vi "Vision.vi"() -> ()   [LabVIEW 2021]
doc: "Main VI for the vision algorithm. Shows camera footage and extracts ball and plate position, that are then written on the myRIO microcontroller to be used by other programs. Refresh rate of coordinates is 17ms"
uses:
  <vilib>/Platform/TimedLoop/XDataNode/timing_clust.ctl
  <vilib>/Platform/TimedLoop/XDataNode/nitl_modes.ctl
  <vilib>/Platform/TimedLoop/XDataNode/wakeup.ctl
  <vilib>/Platform/TimedLoop/XDataNode/XDataNode.xnode
  <vilib>/Platform/TimedLoop/XDataNode/XDNodeRunTimeDep.lvlib
panel:
  in  "Exposure::Value":dbl=1.0 min=0.0625 max=32.0
  in  "Exposure::Mode":u32(ring)=2 items=["Auto"=1, "Manual"=2]
  in  "error in":errorcluster
  out "Ball Coordinates":sgl[](array[numeric])
  out "Plate coordinates":sgl[](array[numeric])
  out "error out":errorcluster
  out "Frame Rate":dbl
  in  "Stop (F)":bool
  out "Image Out":T1(plugin-control)
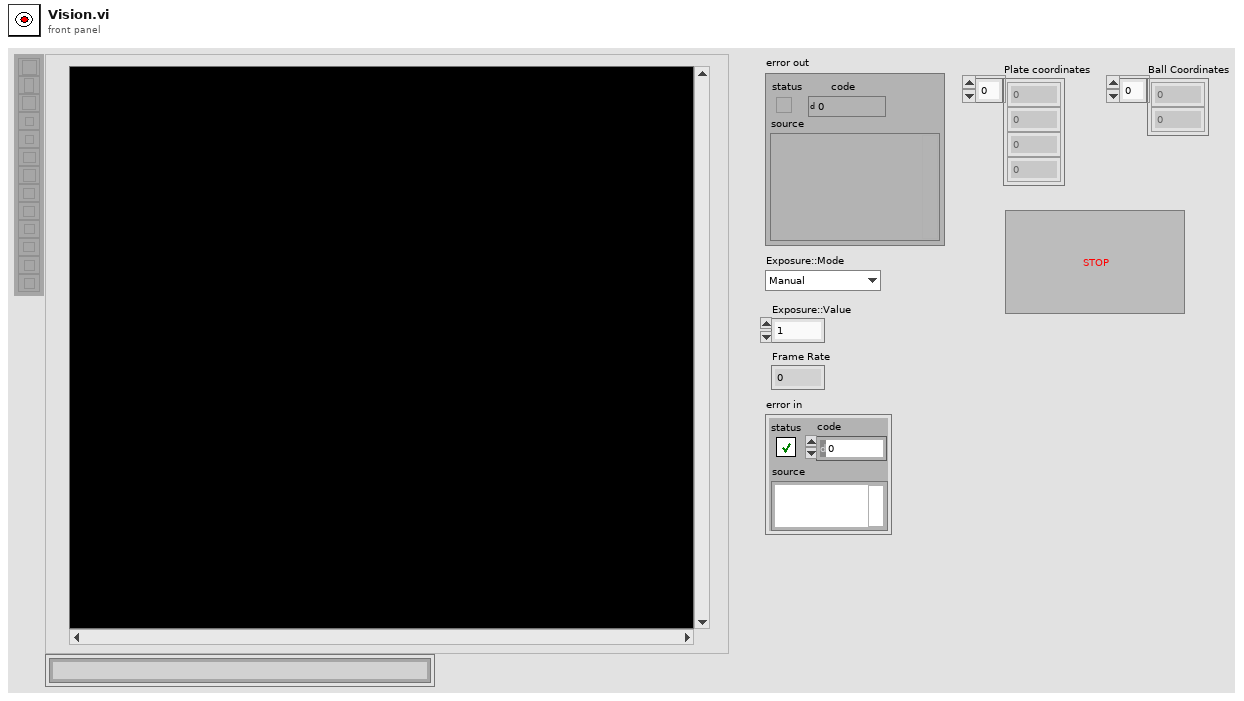
[diagram p1: front panel]
types:
  T1 = typedef "IMAQ Image.ctl" = refnum<image>
  T2 = typedef "XDNodeRunTimeDep.lvlib/timing_clust.ctl" = cluster{"Expected End [f-1]":u64, "Actual End [f-1]":u64, "Finished Late? [f-1]":bool, "Expected End [i-1]":u64, "Actual End [i-1]":u64, "Finished Late? [i-1]":bool, "Expected Start [i]":u64, "Actual Start [i]":u64, "Expected Start [f]":u64, "Actual Start [f]":u64, "Source Name":string, "Structure Name":string, "Period":i64, "Deadline":i64, "Offset":i64, "Start":i64, "Priority":i32, "Timeout":i32, "Mode":T3, "Wakeup Reason":T4, "Error":errorcluster, "Source Type":string, "Secondary Source Type":string, "Global End Time":u64, "Global Start Time":u64, "Frame Duration":u64, "Iteration Duration":u64, "Assigned CPU":i32, "I/O Scan Engine Mode":u32}
  T3 = typedef "XDNodeRunTimeDep.lvlib/nitl_modes.ctl" = enum32{"No Change", "Process missed periods, maintain original phase", "Discard missed periods, maintain original phase", "Process missed periods, ignore original phase", "Discard missed periods, ignore original phase"}
  T4 = typedef "XDNodeRunTimeDep.lvlib/wakeup.ctl" = enum32{"Normal", "Aborted", "Asynchronous wakeup", "Timing source error", "Timed loop error", "Timeout"}
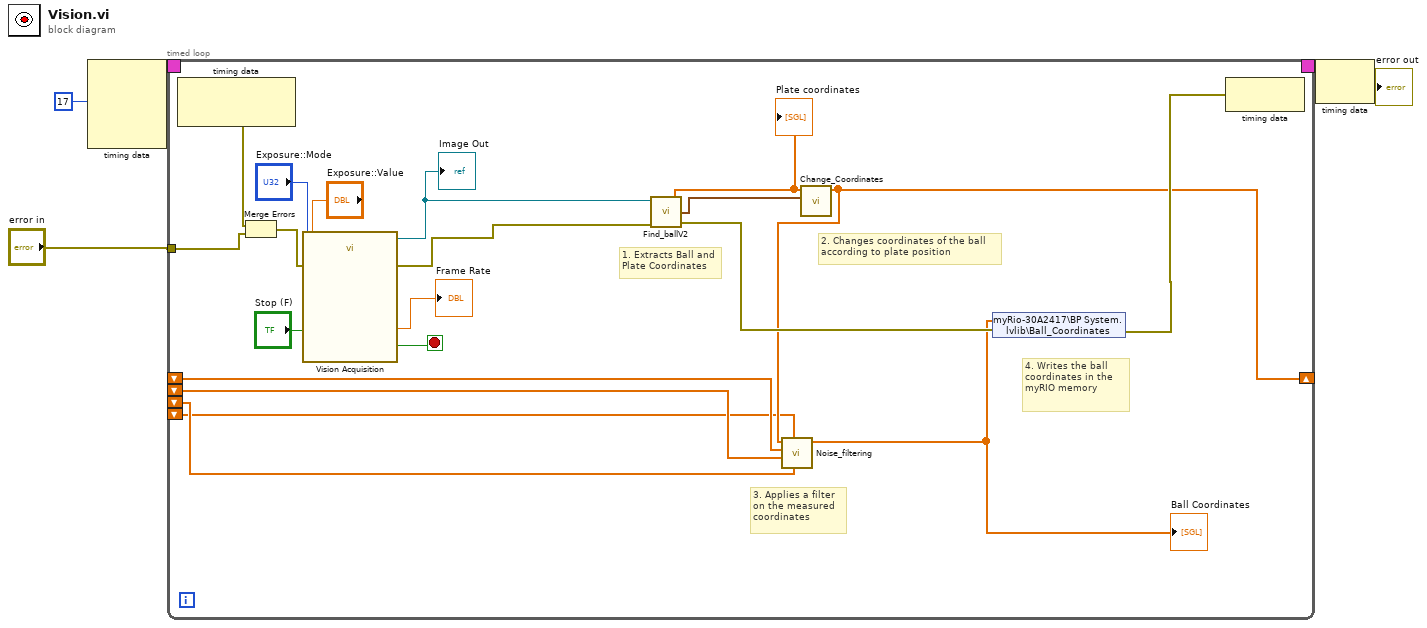
[diagram p0: block diagram]
diagram:
  n1 = node-c288(i64 17 ("Period")) -> (w5:T2)  [unwired: 3 in]
  n2 = timed-loop {
    timing: w5 -> [_]
    timing-out: [_] -> w4
    tunnel: "error in" -> [w15]
    shift-right: [w11] -> _
    shift-left: _ -> [w10]
    shift-left: _ -> [w9]
    shift-left: _ -> [w8]
    shift-left: _ -> [w7]
    stop <- w24 stop-if-true
    # "4. Writes the ball coordinates in the myRIO memory"
    # "2. Changes coordinates of the ball\naccording to plate position"
    # "1. Extracts Ball and\nPlate Coordinates"
    # "3. Applies a filter\non the measured \ncoordinates"
    n3 = node-c288() -> (w16:errorcluster)  [unwired: 1 in, 1 out]
    n4 = Merge Errors(w16, w15) -> (w14:errorcluster)
    n5 = call "Vision Acquisition"("Exposure::Mode"="Exposure::Mode", "Exposure::Value"="Exposure::Value", "Stop (F)"="Stop (F)", "error in"=w14) -> ("Image Out"=w22:T1, "Frame Rate"=→"Frame Rate":dbl, "Stopped"=w24:bool, "error out"=w18:errorcluster)  [unwired: 20 in]
    "Image Out" <- w22
    n6 = call "Find_ballV2.vi"("Image In"=w22, "error in"=w18) -> ("Plate coordinates"=w20:sgl[], "Ball Coordinates"=w21:cluster{"x":sgl, "y":sgl}, "error out"=w19:errorcluster)  [unwired: 2 in, 1 out]
    "Plate coordinates" <- w20
    n7 = call "Change_Coordinates.vi"("Ball Coordinates"=w21, "Plate coordinates"=w20) -> ("Array"=w11:sgl[])  [unwired: 9 in]
    n8 = call "Noise_filtering.vi"("Array 3"=w8, "Array in"=w7, "Array 4"=w9, "Array 5"=w10, "Array 6"=w11) -> ("Array out"=w6:dbl[])  [unwired: 6 in]
    "Ball Coordinates" <- w6
    n9 = shared-variable "myRio-30A2417\\BP System.lvlib\\Ball_Coordinates"(w6, error in=w19) -> (error out=w17:errorcluster)
    n10 = node-c288(w17) -> ()  [unwired: 1 out]
  }
  n11 = node-c288(w4) -> (→"error out":errorcluster)
